vi "Queues.vi"() -> ()   [LabVIEW 2019]
doc: "Use this template to build a producer/consumer design pattern. Use this template when you need to execute a process, such as data analysis, when a data source, such as a triggered acquisition, produces data at an uneven rate and you need to execute the process when the data becomes available."
panel:
  out "elements":string[](array[string])
  out "Ciclo Status Queue":i32
  out "Tank":i32(slide) scale=0.0..100.0
  in  "stop":bool
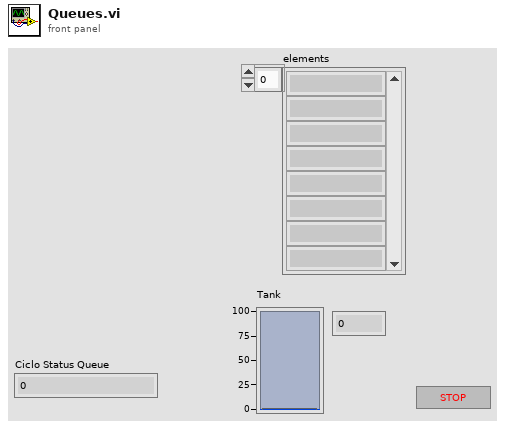
[diagram p1: front panel]
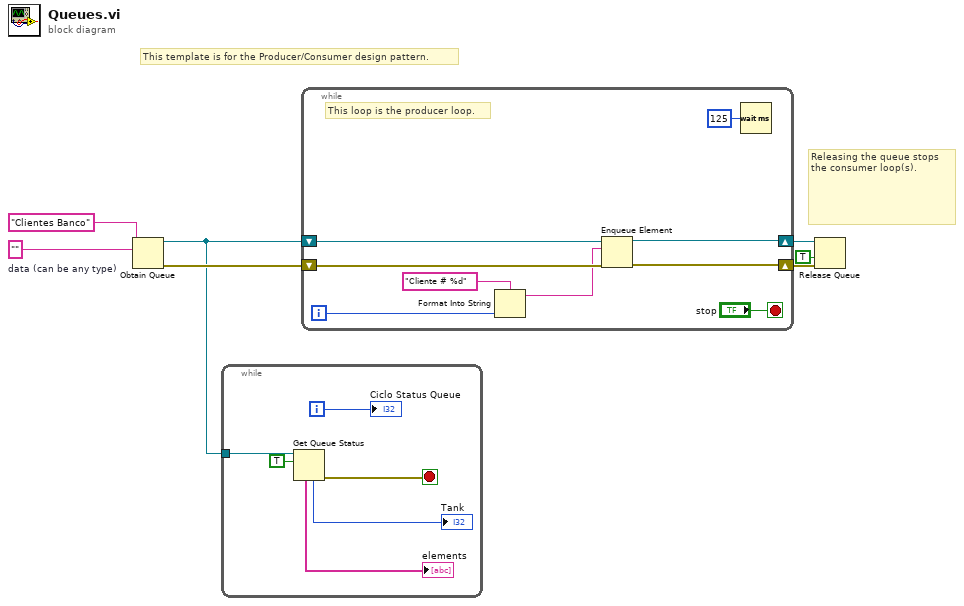
[diagram p0: block diagram]
diagram:
  w4 = ""  # data (can be any type)
  # "Releasing the queue stops the consumer loop(s)."
  # "This template is for the Producer/Consumer design pattern."
  n1 = Obtain Queue(name (unnamed)="Clientes Banco", element data type=w4) -> (queue out=w1:refnum<queue>, error out=w7:errorcluster)  [unwired: 3 in, 1 out]
  n2 = while {
    tunnel: w1 -> [w12]
    i -> [w10]
    stop <- w13 stop-if-true
    n3 = Get Queue Status(queue=w12, return elements? (F)=TRUE) -> (error out=w13:errorcluster, # elements in queue=→"Tank":i32, elements=→"elements":string[])  [unwired: 1 in, 5 out]
    "Ciclo Status Queue" <- w10
  }
  n4 = while {
    shift-right: [w21] -> w6
    shift-left: w7 -> [w22]
    shift-right: [w18] -> w5
    shift-left: w1 -> [w19]
    i -> [w16]
    stop <- "stop" stop-if-true
    # "This loop is the producer loop."
    n5 = Format Into String(format string="Cliente # %d", w16) -> (resulting string=w15:string)  [unwired: 2 in, 1 out]
    n6 = Enqueue Element(queue=w19, element=w15, error in (no error)=w22) -> (queue out=w18:refnum<queue>, error out=w21:errorcluster)  [unwired: 1 in, 1 out]
    n7 = Wait (ms)(milliseconds to wait=u32 125) -> ()  [unwired: 1 out]
  }
  n8 = Release Queue(queue=w5, force destroy? (F)=TRUE, error in (no error)=w6) -> ()  [unwired: 3 out]
